vi "EasyXML Options - Unflatten Data.vi"(8 "error in":errorcluster, 11 "EasyXML Options in":T4) -> (0 "error out":errorcluster, 3 "Easy XML Options out":T1)   [LabVIEW 2011]
uses:
  Support/Type Defs/EasyXML Options.ctl
  EasyXML Options - Data Cluster.ctl
  EasyXML Options - Type Formatting Cluster.ctl
  Support/Type Defs/Formatting Data Type -- Enum.ctl
panel:
  in  "Case Constant\n(See Context Help)":bool
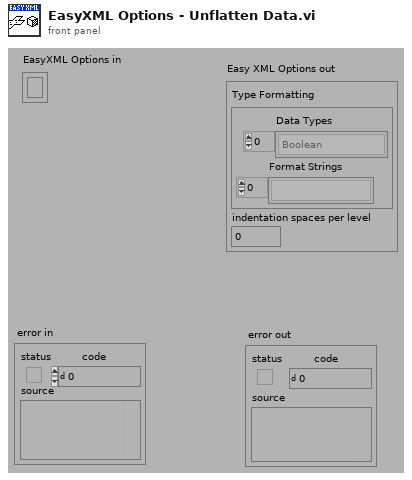
[diagram p1: front panel]
types:
  T1 = typedef "EasyXML Options - Data Cluster.ctl" = cluster{"Type Formatting":T2, "indentation spaces per level":i32}
  T2 = typedef "EasyXML Options - Type Formatting Cluster.ctl" = cluster{"Data Types":T3[], "Format Strings":string[]}
  T3 = typedef "Formatting Data Type -- Enum.ctl" = enum16{"<unknown>", "Cluster", "Array", "String", "Path", "Boolean", "Time Stamp", "Enum", "Numeric - EXT", "Numeric - DBL", "Numeric - SGL", "Numeric - I64", "Numeric - I32", "Numeric - I16", "Numeric - I8", "Numeric - U64", "Numeric - U32", "Numeric - U16", "Numeric - U8", "Numeric - CXT", "Numeric - CDB", "Numeric - CSG", "VISA Resource"}
  T4 = typedef "EasyXML Options.ctl" = cluster{"Data":variant}
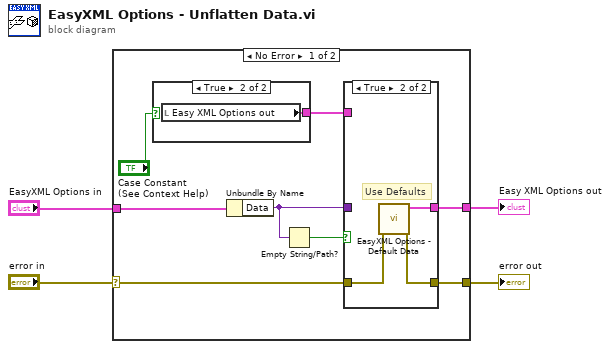
[diagram p0: block diagram]
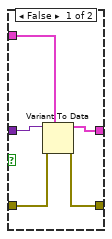
[diagram p2: hidden frame]
diagram:
  n1 = case shown="No Error" "error in" {
    selector: "error in" -> [w7 w22]
    tunnel: "EasyXML Options in" -> [w11 _]
    tunnel: [w10 w22] -> w3
    tunnel: [w9 _] -> w2
    frame No Error {
      n2 = case shown="True" "Case Constant\n(See Context Help)" {
        tunnel: [_ w21] -> w12
        frame False {
        }
        frame True {
          n3 = local read "Easy XML Options out"() -> (w21:T1)
        }
      }
      n4 = Unbundle By Name(w11) -> ("Data"=w6:variant)
      n5 = Empty String/Path?(string/path=w6) -> (empty?=w5:bool)
      n6 = case shown="True" w5 {
        tunnel: w12 -> [w17 _]
        tunnel: [w16 w18] -> w10
        tunnel: [w15 w20] -> w9
        tunnel: w7 -> [w14 w19]
        tunnel: w6 -> [w13 _]
        frame False {
          n7 = Variant To Data(error in=w14, type=w17, Variant=w13) -> (data=w15:T1, error out=w16:errorcluster)
        }
        frame True {
          # "Use Defaults"
          n8 = call "EasyXML Options - Default Data.vi"("error in"=w19) -> ("error out"=w18:errorcluster, "Default Easy XML Options"=w20:T1)  [unwired: 9 in]
        }
      }
    }
    frame Error {
    }
  }
  "Easy XML Options out" <- w2
  "error out" <- w3
